vi "Configure Reference Offset.vi"(6 "Enable Amps Reference (F: Disable)":bool, 7 "Reference Value (0.0000000E+0)":dbl format="%.7e", 8 "error in (no error)":errorcluster, 9 "Enable Reference (F: Disable)":bool, 10 "Measurement Function (0: Voltage)":i32(ring) items=["Voltage", "Current", "Resistance", "Charge"], 11 "VISA resource name":refnum<visa-resource-name>) -> (0 "error out":errorcluster, 3 "VISA resource name out":refnum<visa-resource-name>)   [LabVIEW 2020, in "Keithley 6517.lvlib"]
doc: "Configures the offset settings for the measurement functions (Voltage, Current, Resistance and Charge).\n\nNote:\nThe specified measurement should be enabled from <b>Configure Measurement Function.vi</b>.\n\nThis VI is <B>NOT</B> compatible with model <B>6514</B>."
uses:
  <instrlib>/Keithley 6517/Keithley 6517.lvlib
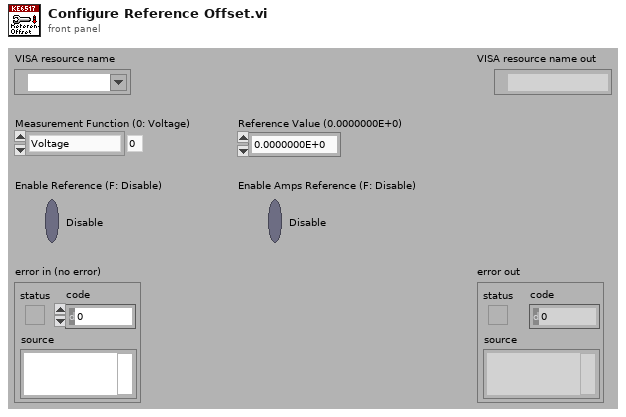
[diagram p1: front panel]
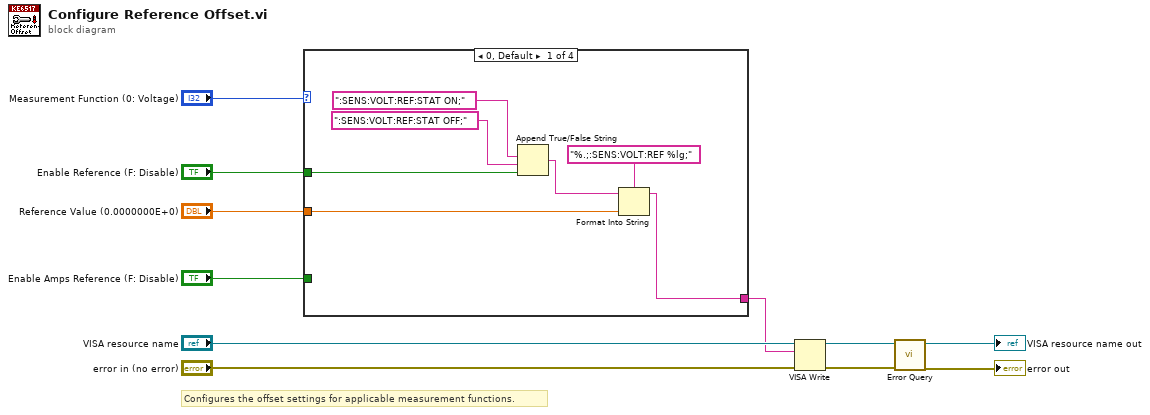
[diagram p0: block diagram]
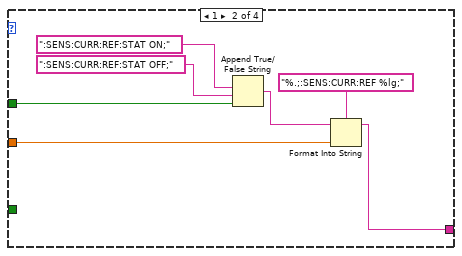
[diagram p2: hidden frame]
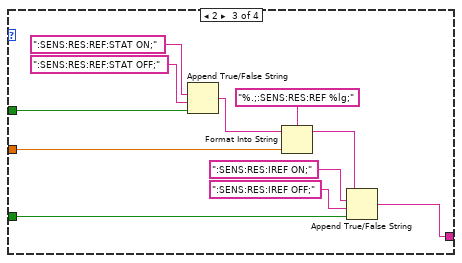
[diagram p3: hidden frame]
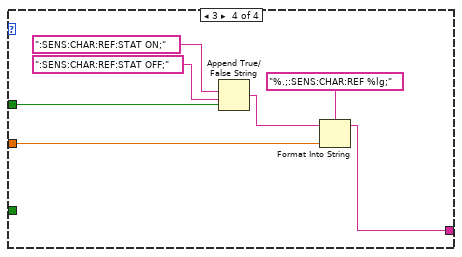
[diagram p4: hidden frame]
diagram:
  # "Configures the offset settings for applicable measurement functions."
  n1 = case shown="0, Default" "Measurement Function (0: Voltage)" {
    tunnel: "Enable Reference (F: Disable)" -> [w14 w21 w32 w39]
    tunnel: "Reference Value (0.0000000E+0)" -> [w13 w20 w31 w38]
    tunnel: "Enable Amps Reference (F: Disable)" -> [_ _ w28 _]
    tunnel: [w12 w19 w26 w37] -> w1
    frame 0, Default {
      n2 = Append True/False String(1:w14, 2:":SENS:VOLT:REF:STAT OFF;", 3:":SENS:VOLT:REF:STAT ON;") -> (0:w17:string)  [unwired: 1 in]
      n3 = Format Into String(format string="%.;:SENS:VOLT:REF %lg;", initial string=w17, w13) -> (resulting string=w12:string)  [unwired: 1 in, 1 out]
    }
    frame 1 {
      n4 = Append True/False String(1:w21, 2:":SENS:CURR:REF:STAT OFF;", 3:":SENS:CURR:REF:STAT ON;") -> (0:w25:string)  [unwired: 1 in]
      n5 = Format Into String(format string="%.;:SENS:CURR:REF %lg;", initial string=w25, w20) -> (resulting string=w19:string)  [unwired: 1 in, 1 out]
    }
    frame 2 {
      n6 = Append True/False String(1:w32, 2:":SENS:RES:REF:STAT OFF;", 3:":SENS:RES:REF:STAT ON;") -> (0:w30:string)  [unwired: 1 in]
      n7 = Format Into String(format string="%.;:SENS:RES:REF %lg;", initial string=w30, w31) -> (resulting string=w27:string)  [unwired: 1 in, 1 out]
      n8 = Append True/False String(1:w28, 2:":SENS:RES:IREF OFF;", 3:":SENS:RES:IREF ON;", 4:w27) -> (0:w26:string)
    }
    frame 3 {
      n9 = Append True/False String(1:w39, 2:":SENS:CHAR:REF:STAT OFF;", 3:":SENS:CHAR:REF:STAT ON;") -> (0:w42:string)  [unwired: 1 in]
      n10 = Format Into String(format string="%.;:SENS:CHAR:REF %lg;", initial string=w42, w38) -> (resulting string=w37:string)  [unwired: 1 in, 1 out]
    }
  }
  n11 = VISA Write(VISA resource name="VISA resource name", write buffer=w1, error in (no error)="error in (no error)") -> (VISA resource name out=w9:refnum<visa-resource-name>, error out=w8:errorcluster)  [unwired: 1 out]
  n12 = call <instrlib>:"Error Query.vi"("error in (no error)"=w8, "VISA resource name"=w9) -> ("error out"=→"error out":errorcluster, "VISA resource name out"=→"VISA resource name out":refnum<visa-resource-name>)  [unwired: 6 in, 2 out]
